vi "Get Section Name.vi"(11 "Dummy Usage in":refnum<class "Dummy Usage.lvclass">) -> (2 "Section":string, 3 "Dummy Usage out":refnum<class "Dummy Usage.lvclass">)   [LabVIEW 2019, in "Electronic Datasheet.lvlib" / "Dummy Usage.lvclass"]
uses:
  Dummy Usage.lvclass
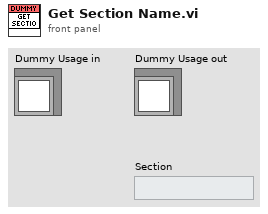
[diagram p1: front panel]
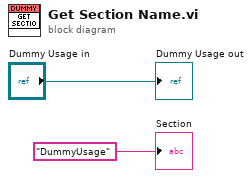
[diagram p0: block diagram]
diagram:
  "Dummy Usage out" <- "Dummy Usage in"
  "Section" <- "DummyUsage" ("Section")
